vi "RandDirVec.vi"(10 "Length":dbl, 11 "Rays":u32) -> (3 "DirVecs":dbl[][](array[numeric]))   [LabVIEW 2014]
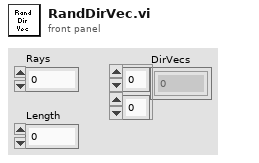
[diagram p1: front panel]
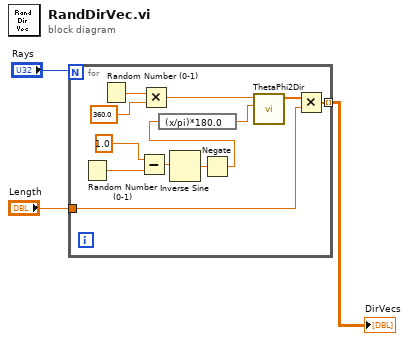
[diagram p0: block diagram]
diagram:
  n1 = for {
    N: "Rays" -> [_]
    tunnel: [w11] -> w2 mode=indexing
    tunnel: "Length" -> [w4]
    n2 = Random Number (0-1)() -> (number: 0 to 1=w5:dbl)
    n3 = Random Number (0-1)() -> (number: 0 to 1=w15:dbl)
    n4 = Subtract(x=1.0 ("y"), y=w5) -> (x-y=w9:dbl)
    n5 = Multiply(x=w15, y=360.0) -> (x*y=w13:dbl)
    n6 = Inverse Sine(1:w9) -> (0:w8:dbl)
    n7 = Negate(x=w8) -> (-x=w6:dbl)
    n8 = expression code="(x/pi)*180.0" ("radians to degrees")(w6) -> (w7:dbl)
    n9 = call "ThetaPhi2Dir.vi"("Phi"=w7, "Theta"=w13) -> ("Dir"=w12:dbl[])  [unwired: 9 in]
    n10 = Multiply(x=w12, y=w4) -> (x*y=w11:dbl[])
  }
  "DirVecs" <- w2
